vi "loadConfig.vi"(8 "error in (no error)":errorcluster caption="错误输入（无错误）", 10 "calFilePath":string, 11 "abstractVNA 输入":refnum<class "abstractVNA.lvclass"> caption="DNL_LabVIEW Object in") -> (0 "error out":errorcluster caption="错误输出", 3 "abstractVNA 输出":refnum<class "abstractVNA.lvclass"> caption="DNL_LabVIEW Object out")   [LabVIEW 2011, in "abstractVNA.lvclass"]
uses:
  abstractVNA.lvclass
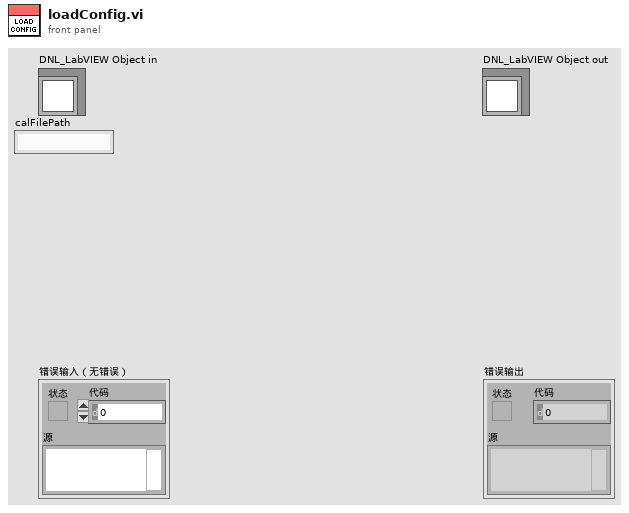
[diagram p1: front panel]
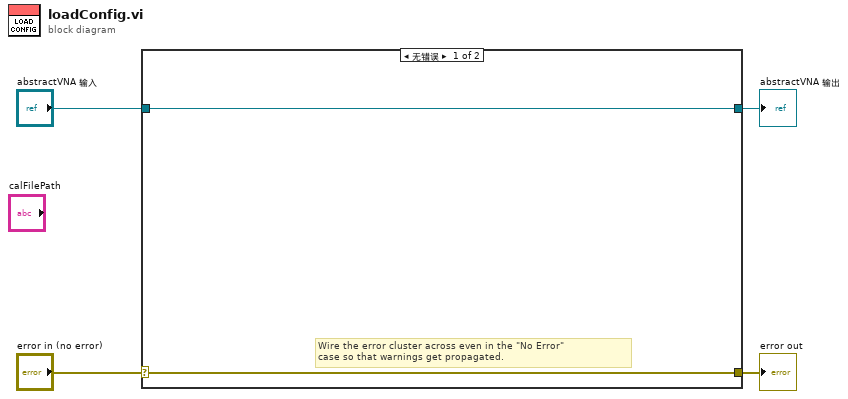
[diagram p0: block diagram]
diagram:
  n1 = case shown="无错误" "error in (no error)" {
    selector: "error in (no error)" -> [w5 w8]
    tunnel: [w5 w8] -> w3
    tunnel: [w6 w7] -> w1
    tunnel: "abstractVNA 输入" -> [w6 w7]
    frame No Error {
      # "Wire the error cluster across even in the \"No Error\"\ncase so that warnings get propagated."
    }
    frame Error {
    }
  }
  "error out" <- w3
  "abstractVNA 输出" <- w1
